vi "pr1c2.vi"() -> ()   [LabVIEW 2013]
uses:
  <vilib>/Utility/error.llb/DialogType.ctl
  <vilib>/DAQmx/write.llb/DAQmx Write (Digital Wfm 1Chan NSamp).vi
  <vilib>/DAQmx/create/channels.llb/DAQmx Create Channel (CO-Pulse Generation-Frequency).vi
  <vilib>/DAQmx/configure/timing.llb/DAQmx Timing (Implicit).vi
  <vilib>/Waveform/DWDTOps.llb/DWDT Boolean Array to Digital.vi
  <vilib>/DAQmx/create/channels.llb/DAQmx Create Channel (DO-Digital Output).vi
  <vilib>/DAQmx/configure/timing.llb/DAQmx Timing (Sample Clock).vi
  <vilib>/Waveform/DWDTOps.llb/DWDT Uncompress Digital.vi
  <vilib>/DAQmx/miscellaneous.llb/DAQmx Fill In Error Info.vi
panel:
  in  "lines":tag
  in  "Duty Cycle":dbl=1.0 min=0.0 max=100.0 step=0.01 format="%#_5g"
  out "Frecuencia PWM":dbl
  out "Frecuencia de la base de tiempos (Hz)":dbl=1.0 format="%.8f"
  in  "Numero de Pulsos por muestreo (N)":i32=1
  in  "Periodo de muestreo":dbl=1.0 format="%.8f"
  in  "Counter":tag="Dev1/ctr0"
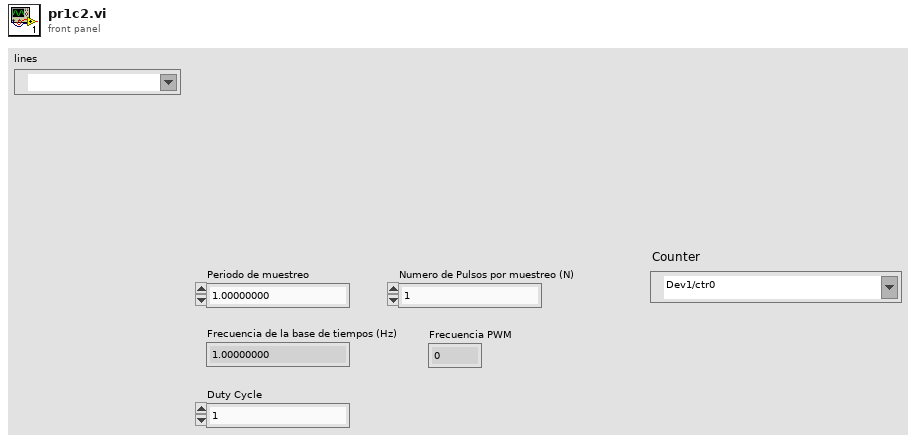
[diagram p1: front panel]
types:
  T1 = typedef "DialogType.ctl" = u16
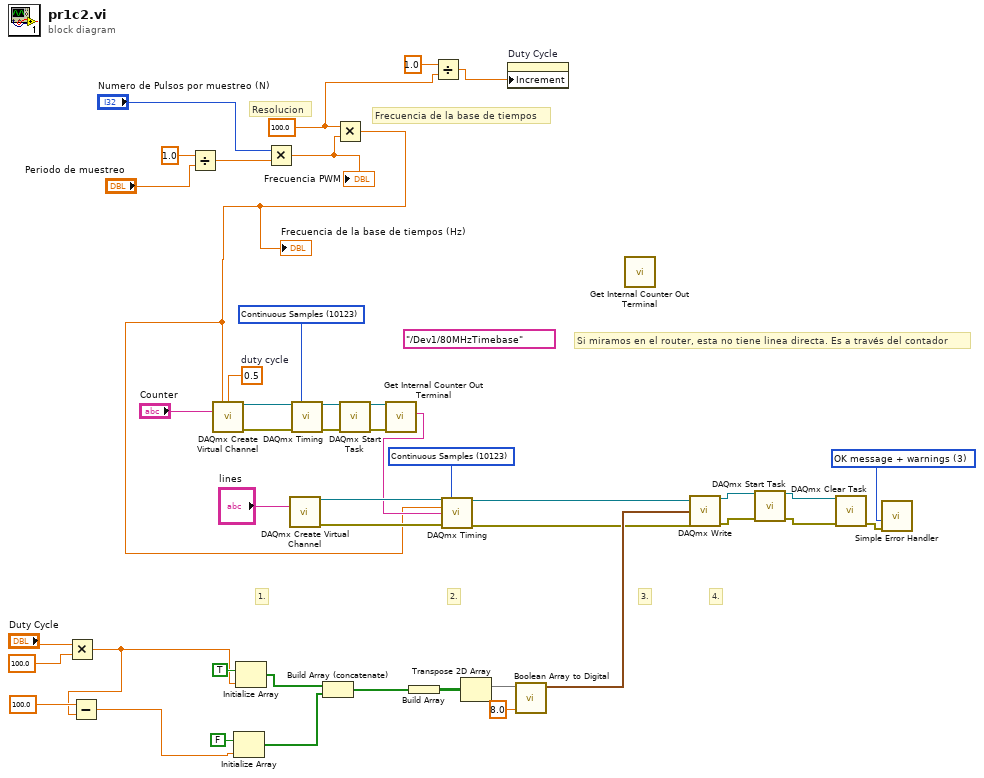
[diagram p0: block diagram]
diagram:
  w24 = 100.0 ("x")
  (unwired) tag "/Dev1/80MHzTimebase" ("source")
  w35 = 0.5  # duty cycle
  w39 = 10123 items=["Finite Samples"=10178, "Continuous Samples"=10123, "Hardware Timed Single Point"=12522] ("sample mode")
  w41 = 10123 items=["Finite Samples"=10178, "Continuous Samples"=10123, "Hardware Timed Single Point"=12522] ("sample mode")
  w44 = T1 3 items=["no dialog", "OK message", "continue or stop message", "OK message + warnings", "continue/stop + warnings"] ("type of dialog (OK msg:1)")
  # "Resolucion"
  # "Frecuencia de la base de tiempos"
  # "Si miramos en el router, esta no tiene linea directa. Es a través del contador"
  # "4."
  # "3."
  # "2."
  # "1."
  n1 = Multiply(x="Duty Cycle", y=100.0) -> (x*y=w16:dbl)
  n2 = Subtract(x=100.0, y=w16) -> (x-y=w15:dbl)
  n3 = Divide(x=1.0, y="Periodo de muestreo") -> (x/y=w29:dbl)
  n4 = Initialize Array(FALSE, w15) -> (w19:bool[])
  n5 = Initialize Array(TRUE, w16) -> (w21:bool[])
  n6 = Multiply(x="Numero de Pulsos por muestreo (N)", y=w29) -> (x*y=w27:dbl)
  "Frecuencia PWM" <- w27
  n7 = call-poly <vilib>:"DAQmx Create Virtual Channel.vi"("lines"="lines") -> ("task out"=w43:refnum<k21>, "error out"=w42:errorcluster)  [unwired: 13 in]
  n8 = Build Array (concatenate)(w21, w19) -> (w11:bool[])
  n9 = Multiply(x=w24, y=w27) -> (x*y=w9:dbl)
  "Frecuencia de la base de tiempos (Hz)" <- w9
  n10 = call-poly <vilib>:"DAQmx Create Virtual Channel.vi"("frequency"=w9, "duty cycle"=w35, "counter"="Counter") -> ("task out"=w32:refnum<k21>, "error out"=w34:errorcluster)  [unwired: 6 in, 5 out]
  n11 = call-poly <vilib>:"DAQmx Timing.vi"("task/channels in"=w32, "sample mode"=w39, "error in"=w34) -> ("task out"=w38:refnum<k21>, "error out"=w37:errorcluster)  [unwired: 2 in, 9 out]
  n12 = call <vilib>:"DAQmx Start Task.vi"("task/channels in"=w38, "error in"=w37) -> ("task out"=w33:refnum<k21>, "error out"=w36:errorcluster)  [unwired: 12 out]
  n13 = call "Get Internal Counter Out Terminal.vi"("error in (no error)"=w36, "task in"=w33) -> ("internal counter out"=w14:string)  [unwired: 7 in, 2 out]
  n14 = Build Array(w11) -> (w10:bool[][])
  n15 = Divide(x=1.0, y=w24) -> (x/y=w25:dbl)
  n16 = call-poly <vilib>:"DAQmx Timing.vi"("task/channels in"=w43, "sample mode"=w41, "rate"=w9, "source"=w14, "error in"=w42) -> ("task out"=w8:refnum<k21>, "error out"=w7:errorcluster)  [unwired: 9 in]
  n17 = Transpose 2D Array(2D array=w10) -> (transposed array=w12:bool[][])
  n18 = property on="Duty Cycle" class="DigNum (strict)"("Increment"=w25) -> ()  [unwired: 2 in, 2 out]
  n19 = call-poly <vilib>:"Boolean Array to Digital.vi"("sample rate"=8.0, "boolean array"=w12) -> ("digital waveform"=w13:digitalwaveform)  [unwired: 8 in, 1 out]
  n20 = call "Get Internal Counter Out Terminal.vi"() -> ()  [unwired: 9 in, 3 out]
  n21 = call-poly <vilib>:"DAQmx Write.vi"("task/channels in"=w8, "data"=w13, "error in"=w7) -> ("task out"=w5:refnum<k21>, "error out"=w6:errorcluster)  [unwired: 10 in, 1 out]
  n22 = call <vilib>:"DAQmx Start Task.vi"("task/channels in"=w5, "error in"=w6) -> ("task out"=w4:refnum<k21>, "error out"=w3:errorcluster)  [unwired: 12 in]
  n23 = call <vilib>:"DAQmx Clear Task.vi"("task in"=w4, "error in"=w3) -> ("error out"=w45:errorcluster)  [unwired: 13 in]
  n24 = call <vilib>:"Simple Error Handler.vi"("type of dialog (OK msg:1)"=w44, "error in (no error)"=w45) -> ()  [unwired: 3 in, 5 out]
